vi "FibrePhotometry_AutoOptimization.vi"() -> ()   [LabVIEW 2017]
panel:
  out "Current 470 nm inputs":dbl
  out "Current 405nm input":dbl
  in  "DataFolder":path=path "C:/DATA/test"
  in  "RecDur4EachCondition (min)":dbl=1.0
  in  "Freq (Hz)":dbl=40.0
  in  "470nm inputs (V)":dbl[](array[numeric])=[0.5, 1.0, 1.5, 2.0]
  in  "405nm inputs (V)":dbl[](array[numeric])=[0.5, 1.0, 1.5, 2.0]
  # "Automatic Optimization for LED input level"
  # "Instruction\n1. set parameters, in particular inputs and DataFolder\n* DataFolder should be a separate folder from the main folder where you will save data for your main data, such as sleep rec.\n2. run"
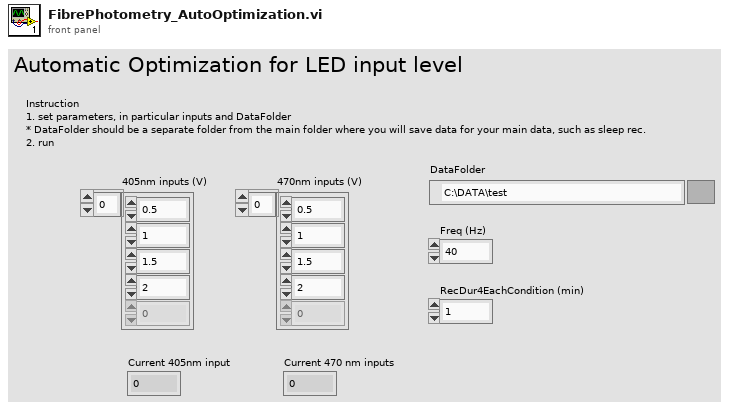
[diagram p1: front panel]
types:
  T1 = enum16{"open", "replace", "create", "open or create", "replace or create", "replace or create with confirmation"}
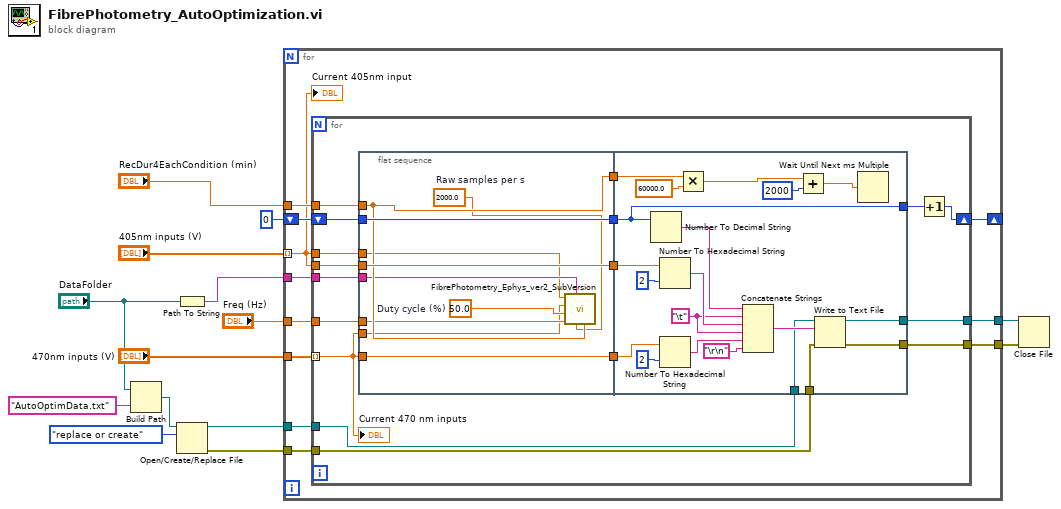
[diagram p0: block diagram]
diagram:
  n1 = Build Path(base path="DataFolder", name or relative path="AutoOptimData.txt") -> (appended path=w6:path)
  n2 = Path To String(path="DataFolder") -> (string=w10:string)
  n3 = Open/Create/Replace File(file path (use dialog)=w6, operation (0:open)=T1."replace or create") -> (refnum out=w4:refnum<file>, error out=w3:errorcluster)  [unwired: 4 in, 1 out]
  n4 = for {
    tunnel: "405nm inputs (V)" -> [w15] mode=indexing
    tunnel: "470nm inputs (V)" -> [w25]
    tunnel: "Freq (Hz)" -> [w16]
    tunnel: "RecDur4EachCondition (min)" -> [w24]
    tunnel: w10 -> [w17]
    shift-right: [w22] -> _
    shift-left: 0 -> [w23]
    tunnel: w4 -> [w21]
    tunnel: w3 -> [w20]
    tunnel: [w19] -> w2
    tunnel: [w18] -> w1
    n5 = for {
      tunnel: w25 -> [w27] mode=indexing
      tunnel: w15 -> [w39]
      tunnel: w24 -> [w34]
      shift-right: [w40] -> w22
      shift-left: w23 -> [w42]
      tunnel: w21 -> [w38]
      tunnel: w20 -> [w37]
      tunnel: [w36] -> w19
      tunnel: [w35] -> w18
      tunnel: w17 -> [w29]
      tunnel: w16 -> [w28]
      tunnel: w15 -> [w26]
      n6 = flat-sequence {
        tunnel: w34 -> [w49]
        tunnel: w27 -> [w50]
        tunnel: w39 -> [w51]
        tunnel: w42 -> [w52]
        tunnel: [w52] -> w33
        tunnel: [w51] -> w32
        tunnel: [w50] -> w31
        tunnel: [w49] -> w30
        tunnel: w29 -> [w47]
        tunnel: w28 -> [w46]
        tunnel: w27 -> [w44]
        tunnel: w26 -> [w43]
        tunnel: [w72] -> w41
        tunnel: w38 -> [w63]
        tunnel: w37 -> [w62]
        tunnel: [w61] -> w36
        tunnel: [w60] -> w35
        tunnel: w33 -> [w72]
        tunnel: w32 -> [w69]
        tunnel: w31 -> [w68]
        tunnel: w30 -> [w57]
        frame #0 {
          w48 = 2000.0  # Raw samples per s
          w45 = 50.0  # Duty cycle (%)
          n7 = call "FibrePhotometry_Ephys_ver2_SubVersion.vi"("RecDur (min)"=w49, "Raw samples per s"=w48, "Dir"=w47, "Frequency"=w46, "Duty cycle (%)"=w45, "470 LED power"=w44, "405 LED Power"=w43) -> ()  [unwired: 5 in]
        }
        frame #1 {
          w66 = "\t"
          n8 = Number To Decimal String(number=w72) -> (decimal integer string=w71:string)  [unwired: 1 in]
          n9 = Number To Hexadecimal String(1:i16 2 ("width (-)"), 2:w69) -> (0:w70:string)
          n10 = Number To Hexadecimal String(1:i16 2 ("width (-)"), 2:w68) -> (0:w67:string)
          n11 = Multiply(x=w57, y=60000.0) -> (x*y=w53:dbl)
          n12 = Concatenate Strings(w71, w66, w70, w66, w67, "\r\n") -> (w64:string)
          n13 = Add(x=w53, y=u32 2000 ("millisecond multiple")) -> (x+y=w55:dbl)
          n14 = Write to Text File(file (use dialog)=w63, text=w64, error in=w62) -> (refnum out=w60:refnum<file>, error out=w61:errorcluster)  [unwired: 1 in, 1 out]
          n15 = Wait Until Next ms Multiple(millisecond multiple=w55) -> ()  [unwired: 1 out]
        }
      }
      n16 = Increment(x=w41) -> (x+1=w40:i32)
      "Current 470 nm inputs" <- w27
    }
    "Current 405nm input" <- w15
  }
  n17 = Close File(refnum=w1, error in=w2) -> ()  [unwired: 2 out]
